vi "Close Session.vi"(8 "error in":errorcluster, 11 "Session HVPS in":refnum<class "Session HVPS.lvclass">) -> (0 "error out":errorcluster, 3 "Session HVPS out":refnum<class "Session HVPS.lvclass">)   [LabVIEW 2013, in "Session HVPS.lvclass"]
uses:
  Session HVPS.lvclass
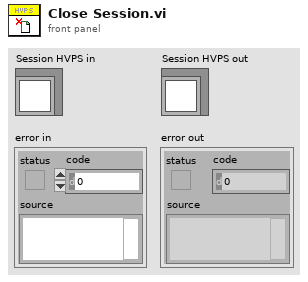
[diagram p1: front panel]
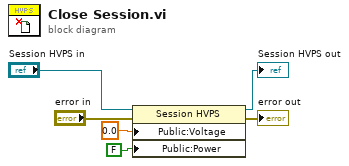
[diagram p0: block diagram]
diagram:
  n1 = property class="Session HVPS"(reference="Session HVPS in", error in="error in", "Public:Voltage"=0.0 ("V"), "Public:Power"=FALSE ("Power")) -> (reference out=→"Session HVPS out":refnum<class "Session HVPS.lvclass">, error out=→"error out":errorcluster)
